vi "CODCr报警信息.vi"(11 "报警簇":T1) -> (3 "CODCR报警信息":string)   [LabVIEW 2016, in "CODCr库.lvlib"]
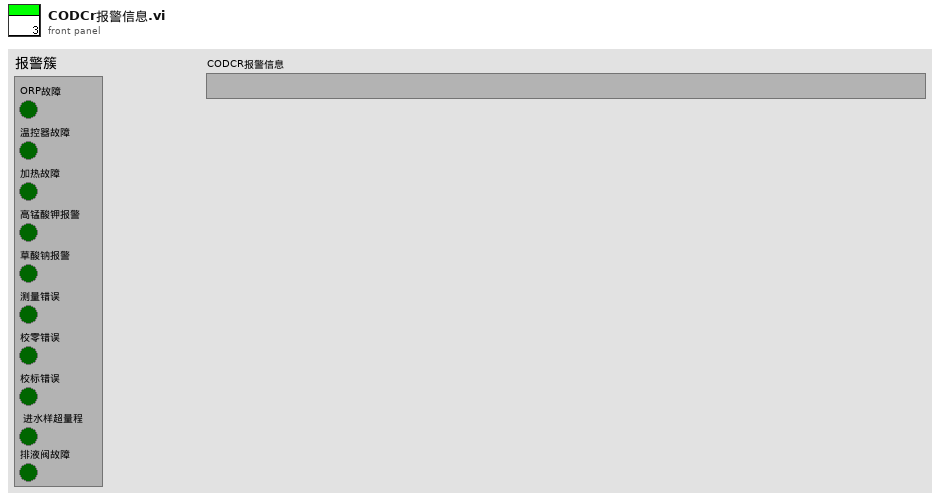
[diagram p1: front panel]
types:
  T1 = cluster{"ORP故障":bool, "温控器故障":bool, "加热故障":bool, "高锰酸钾报警":bool, "草酸钠报警":bool, "测量错误":bool, "校零错误":bool, "校标错误":bool, " 进水样超量程":bool, "排液阀故障":bool}
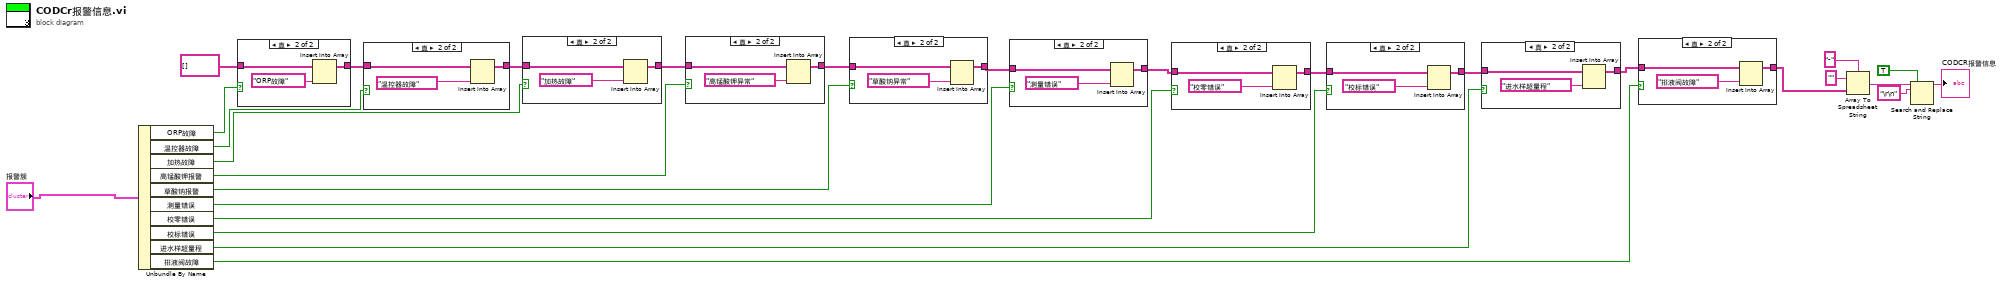
[diagram p0: block diagram]
diagram:
  n1 = Unbundle By Name("报警簇") -> ("ORP故障"=w28:bool, "温控器故障"=w27:bool, "加热故障"=w24:bool, "高锰酸钾报警"=w8:bool, "草酸钠报警"=w7:bool, "测量错误"=w6:bool, "校零错误"=w5:bool, "校标错误"=w4:bool, "进水样超量程"=w3:bool, "排液阀故障"=w2:bool)
  n2 = case shown="真" w28 {
    tunnel: string[] [] -> [w29 w31]
    tunnel: [w29 w30] -> w25
    frame False {
    }
    frame True {
      n3 = Insert Into Array(array=w31, new element="ORP故障" ("组合框")) -> (w30:string[])  [unwired: 1 in]
    }
  }
  n4 = case shown="真" w27 {
    tunnel: w25 -> [w33 w36]
    tunnel: [w33 w35] -> w21
    frame False {
    }
    frame True {
      n5 = Insert Into Array(array=w36, new element="温控器故障" ("组合框")) -> (w35:string[])  [unwired: 1 in]
    }
  }
  n6 = case shown="真" w24 {
    tunnel: w21 -> [w37 w39]
    tunnel: [w37 w40] -> w9
    frame False {
    }
    frame True {
      n7 = Insert Into Array(array=w39, new element="加热故障" ("组合框")) -> (w40:string[])  [unwired: 1 in]
    }
  }
  n8 = case shown="真" w8 {
    tunnel: w9 -> [w41 w43]
    tunnel: [w41 w44] -> w10
    frame False {
    }
    frame True {
      n9 = Insert Into Array(array=w43, new element="高锰酸钾异常" ("组合框")) -> (w44:string[])  [unwired: 1 in]
    }
  }
  n10 = case shown="真" w7 {
    tunnel: w10 -> [w45 w47]
    tunnel: [w45 w48] -> w11
    frame False {
    }
    frame True {
      n11 = Insert Into Array(array=w47, new element="草酸钠异常" ("组合框")) -> (w48:string[])  [unwired: 1 in]
    }
  }
  n12 = case shown="真" w6 {
    tunnel: w11 -> [w49 w51]
    tunnel: [w49 w52] -> w12
    frame False {
    }
    frame True {
      n13 = Insert Into Array(array=w51, new element="测量错误" ("组合框")) -> (w52:string[])  [unwired: 1 in]
    }
  }
  n14 = case shown="真" w5 {
    tunnel: w12 -> [w53 w55]
    tunnel: [w53 w56] -> w15
    frame False {
    }
    frame True {
      n15 = Insert Into Array(array=w55, new element="校零错误" ("组合框")) -> (w56:string[])  [unwired: 1 in]
    }
  }
  n16 = case shown="真" w4 {
    tunnel: w15 -> [w57 w59]
    tunnel: [w57 w60] -> w14
    frame False {
    }
    frame True {
      n17 = Insert Into Array(array=w59, new element="校标错误" ("组合框")) -> (w60:string[])  [unwired: 1 in]
    }
  }
  n18 = case shown="真" w3 {
    tunnel: w14 -> [w61 w63]
    tunnel: [w61 w64] -> w13
    frame False {
    }
    frame True {
      n19 = Insert Into Array(array=w63, new element="进水样超量程" ("组合框")) -> (w64:string[])  [unwired: 1 in]
    }
  }
  n20 = case shown="真" w2 {
    tunnel: w13 -> [w65 w67]
    tunnel: [w65 w68] -> w1
    frame False {
    }
    frame True {
      n21 = Insert Into Array(array=w67, new element="排液阀故障" ("组合框")) -> (w68:string[])  [unwired: 1 in]
    }
  }
  n22 = Array To Spreadsheet String(delimiter (Tab)="-" ("分隔符(Tab)"), array=w1, 3:"" ("格式字符串")) -> (spreadsheet string=w18:string)
  n23 = Search and Replace String(replace all?=TRUE ("替换全部？(F)"), input string=w18, search string="\r\n" ("搜索字符串")) -> (result string=→"CODCR报警信息":string)  [unwired: 5 in, 3 out]
